vi "Scaling(SubVI).vi"(1 "b":dbl, 2 "a":dbl, 3 "X":dbl[](array[numeric])) -> (0 "X'":dbl[](array[numeric]))   [LabVIEW 2017]
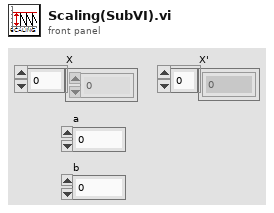
[diagram p1: front panel]
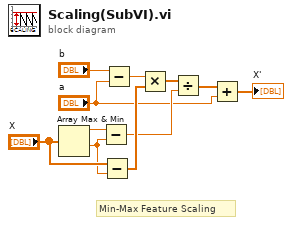
[diagram p0: block diagram]
diagram:
  # "Min-Max Feature Scaling"
  n1 = Array Max & Min(array="X") -> (max value=w11:dbl, min value=w9:dbl)  [unwired: 2 out]
  n2 = Subtract(x=w11, y=w9) -> (x-y=w5:dbl)
  n3 = Subtract(x="X", y=w9) -> (x-y=w6:dbl[])
  n4 = Subtract(x="b", y="a") -> (x-y=w7:dbl)
  n5 = Multiply(x=w7, y=w6) -> (x*y=w4:dbl[])
  n6 = Divide(x=w4, y=w5) -> (x/y=w3:dbl[])
  n7 = Add(x=w3, y="a") -> (x+y=→"X'":dbl[])
